vi "抽取子波形.vi"() -> ()   [LabVIEW 2013]
uses:
  <vilib>/Analysis/NI_AALPro.lvlib
  <vilib>/Analysis/NI_AALBase.lvlib
panel:
  in  "signal type":T1(ring) caption="信号类型"
  out "Original Signal":dbl[](graph)
  out "Extracted Signal":dbl[](graph)
  in  "Stop Button":bool
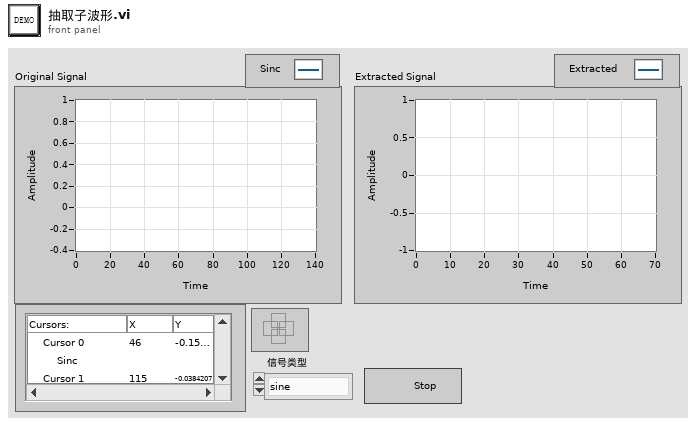
[diagram p1: front panel]
types:
  T1 = enum16{"sine", "cosine", "triangle", "square", "sawtooth", "increasing ramp", "decreasing ramp"}
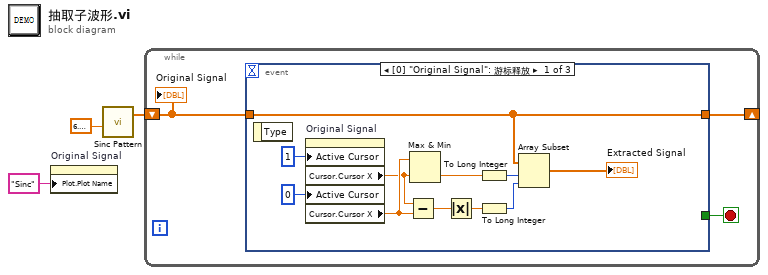
[diagram p0: block diagram]
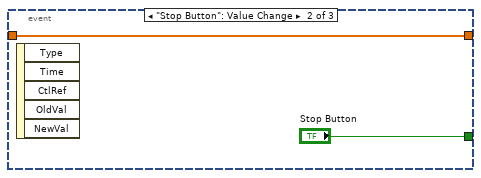
[diagram p2: hidden frame]
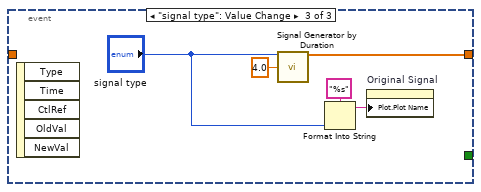
[diagram p3: hidden frame]
diagram:
  n1 = property on="Original Signal" class="WFGraph (严格)"("Plot.Plot Name"="Sinc" ("曲线.曲线名")) -> ()  [unwired: 2 in, 2 out]
  n2 = call <vilib>:"Sinc Pattern.vi"("delay"=6.283185307179586) -> ("Sinc Pattern"=w3:dbl[])  [unwired: 3 in, 1 out]
  n3 = while {
    shift-right: [w5] -> _
    shift-left: w3 -> [w4]
    stop <- w6 stop-if-true
    n4 = event shown="[0] \"Original Signal\": 游标释放" {
      selector: _ -> [_ _ _]
      dyn-events: _ -> [_ _ _]
      timeout: _ -> [_ _ _]
      tunnel: [_ "Stop Button" _] -> w6
      tunnel: [w7 w18 w24] -> w5
      tunnel: w4 -> [w7 w18 _]
      event "Original Signal": Cursor Release {
        n5 = event-data() -> ()  [unwired: 1 in, 1 out]
        n6 = property on="Original Signal" class="WFGraph (严格)"("Active Cursor"=u32 1, "Active Cursor"=u32 0) -> ("Cursor.Cursor X"=w10:dbl, "Cursor.Cursor X"=w11:dbl)  [unwired: 2 in, 2 out]
        n7 = Subtract(x=w10, y=w11) -> (x-y=w13:dbl)
        n8 = Max & Min(x=w11, y=w10) -> (min(x,y)=w9:dbl)  [unwired: 1 out]
        n9 = Absolute Value(x=w13) -> (abs(x)=w12:dbl)
        n10 = To Long Integer(number=w9) -> (32bit integer=w15:i32)
        n11 = To Long Integer(number=w12) -> (32bit integer=w14:i32)
        n12 = Array Subset "Array Subset"(array=w7, index=w15, length=w14) -> (→"Extracted Signal":dbl[])
      }
      event "Stop Button": Value Change {
        n13 = event-data() -> ()  [unwired: 1 in, 5 out]
      }
      event "signal type": Value Change {
        n14 = event-data() -> ()  [unwired: 1 in, 5 out]
        n15 = call <vilib>:"Signal Generator by Duration.vi"("signal type"="signal type", "frequency"=4.0) -> ("signal"=w24:dbl[])  [unwired: 10 in, 3 out]
        n16 = Format Into String(format string="%s" ("格式字符串"), "signal type") -> (resulting string=w21:string)  [unwired: 2 in, 1 out]
        n17 = property on="Original Signal" class="WFGraph (严格)"("Plot.Plot Name"=w21) -> ()  [unwired: 2 in, 2 out]
      }
    }
    "Original Signal" <- w4
  }
